vi "path to cmd argument.vi"(11 "path":path) -> (3 "Array":string[](array[string]))   [LabVIEW 2017]
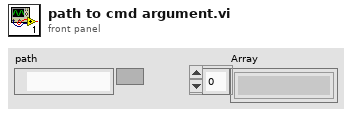
[diagram p1: front panel]
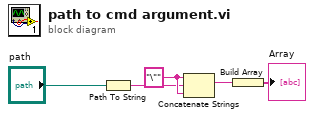
[diagram p0: block diagram]
diagram:
  w3 = "\"" ("string")
  n1 = Path To String(path="path") -> (string=w1:string)
  n2 = Concatenate Strings(w3, w1, w3) -> (w2:string)
  n3 = Build Array(w2) -> (→"Array":string[])
